vi "DAE Radau 5th Order (VIRef).vi"(5 "data":variant, 7 "DAE F(X,X',t)":refnum<vi>, 8 "error in (no error)":errorcluster, 9 "simulation parameters":T1={"initial time"=0.0, "final time"=10.0, "Absolute Tolerance"=[0.001], "Relative Tolerance"=[0.001], "minimum time step"=1e-08, "maximum time step"=1.0, "initial time step"=0.01} {"initial time step" min=0.0; "maximum time step" min=0.0; "minimum time step" min=0.0}, 10 "Initial Derivatives":dbl[](array[numeric]), 11 "Initial Values":dbl[](array[numeric])) -> (0 "error out":errorcluster, 1 "X Derivatives":dbl[][](array[numeric]), 2 "X Values":dbl[][](array[numeric]), 3 "Times":dbl[](array[numeric]))   [LabVIEW 2020, in "NI_DAE.lvlib"]
doc: "Solves differential algebraic equations (DAEs) with initial conditions by using the Radau IIA method. You must manually select the polymorphic instance to use."
uses:
  <vilib>/gmath/NI_DAE.lvlib
  <vilib>/gmath/dae.llb/Radau5_Parameters.ctl
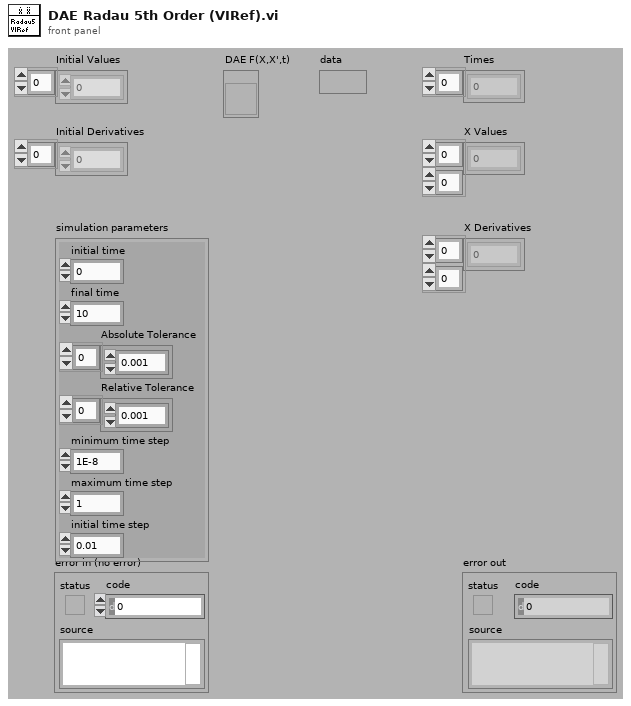
[diagram p1: front panel]
types:
  T1 = typedef "NI_DAE.lvlib/Radau5_Parameters.ctl" = cluster{"initial time":dbl, "final time":dbl, "Absolute Tolerance":dbl[], "Relative Tolerance":dbl[], "minimum time step":dbl, "maximum time step":dbl, "initial time step":dbl}
  T2 = typedef "NI_DAE.lvlib/Radau5_Simulation Data.ctl" = cluster{"initial time":dbl, "final time":dbl, "step size":dbl, "proposed step size":dbl, "max step size":dbl, "min step size":dbl, "Output of T":dbl, "Substep Index":i32, "Timestep Index":i32, "Width":i32, "Absolute tolerance":dbl[], "Relative tolerance":dbl[], "Outputs of Y":dbl[], "Outputs of Y'":dbl[], "Delta":dbl[], "DAE methods":enum16{"default", "Radau IIA"}, "Diag Eval Stage":T3, "step accepted?":bool, "step complete?":bool, "NaN and Inf check?":bool, "First Substep?":bool, "Allow reverse?":bool, "error":errorcluster, "User Jac func?":bool, "Variant":variant, "Index of Y":i8[]}
  T3 = typedef "NI_DAE.lvlib/Radau5_Diag Eval Stage.ctl" = enum16{"Init", "Running", "Final", "End"}
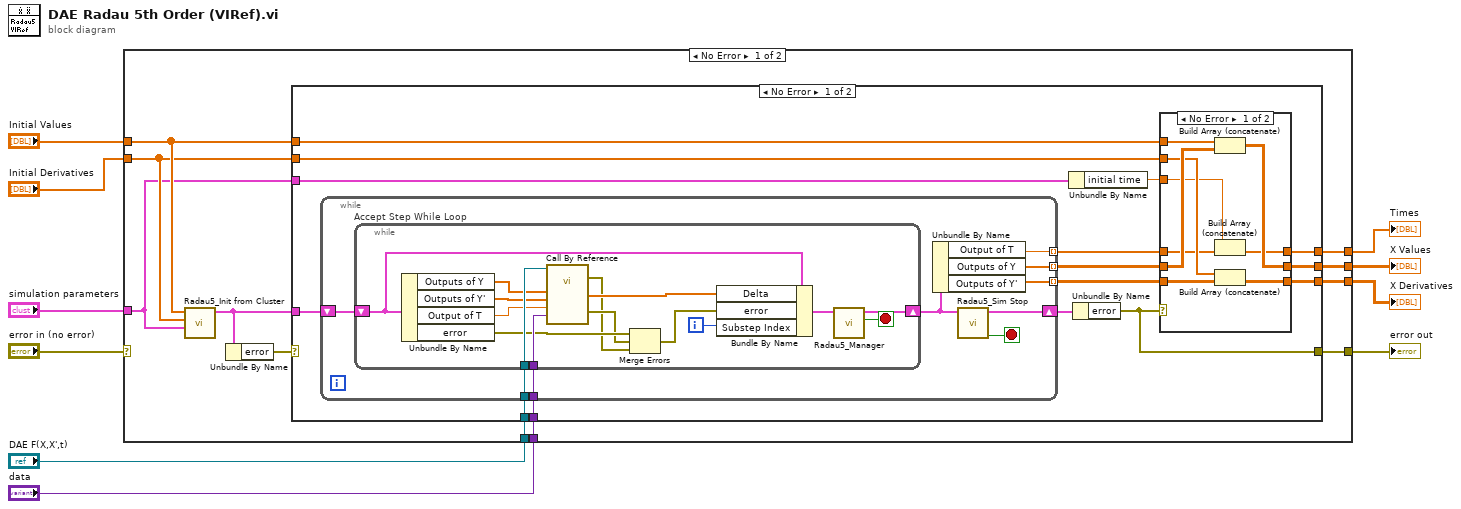
[diagram p0: block diagram]
diagram:
  n1 = case shown="No Error" "error in (no error)" {
    selector: "error in (no error)" -> [_ w71]
    tunnel: [w19 w71] -> w10
    tunnel: [w15 _] -> w9
    tunnel: [w14 _] -> w8
    tunnel: "DAE F(X,X',t)" -> [w21 _]
    tunnel: "data" -> [w20 _]
    tunnel: "Initial Derivatives" -> [w17 _]
    tunnel: "Initial Values" -> [w18 _]
    tunnel: "simulation parameters" -> [w11 _]
    tunnel: [w16 _] -> w1
    frame No Error {
      n2 = call <vilib>:"Radau5_Init from Cluster.vi"("Radau5 Parameters"=w11, "Initial Value Y'"=w17, "Initial Value Y"=w18) -> ("Simulation Data"=w13:T2)  [unwired: 8 in]
      n3 = Unbundle By Name(w13) -> ("error"=w12:errorcluster)
      n4 = case shown="No Error" w12 {
        selector: w12 -> [_ w70]
        tunnel: w21 -> [w35 _]
        tunnel: w20 -> [w34 _]
        tunnel: [w33 w70] -> w19
        tunnel: w18 -> [w29 _]
        tunnel: w17 -> [w28 _]
        tunnel: [w27 _] -> w16
        tunnel: [w26 _] -> w15
        tunnel: [w25 _] -> w14
        tunnel: w13 -> [w24 _]
        tunnel: w11 -> [w23 _]
        frame No Error {
          n5 = while {
            shift-right: [w52] -> w36
            shift-left: w24 -> [w54]
            tunnel: w35 -> [w53]
            tunnel: [w50] -> w30 mode=indexing
            tunnel: [w47] -> w31 mode=indexing
            tunnel: [w49] -> w32 mode=indexing
            tunnel: w34 -> [w46]
            stop <- w51 stop-if-true
            n6 = while "Accept Step While Loop" {
              tunnel: w53 -> [w69]
              shift-right: [w66] -> w48
              shift-left: w54 -> [w68]
              tunnel: w46 -> [w62]
              i -> [w64]
              stop <- w63 stop-if-true
              n7 = Unbundle By Name(w68) -> ("Outputs of Y"=w61:dbl[], "Outputs of Y'"=w60:dbl[], "Output of T"=w59:dbl, "error"=w57:errorcluster)
              n8 = call-by-ref "?"(reference=w69, "data"=w62, "t"=w59, "X'"=w60, "X"=w61) -> (error out=w55:errorcluster, 0:"error out"=w56:errorcluster, "F(X,X',t)"=w65:dbl[])  [unwired: 1 in, 1 out]
              n9 = Merge Errors(w57, w56, w55) -> (w58:errorcluster)
              n10 = Bundle By Name(cluster=w68, "Delta"=w65, "error"=w58, "Substep Index"=w64) -> (w67:T2)
              n11 = call <vilib>:"Radau5_Manager.vi"("Simulation Data In"=w67) -> ("step complete?"=w63:bool, "Simulation Data Out"=w66:T2)  [unwired: 9 in]
            }
            n12 = Unbundle By Name(w48) -> ("Output of T"=w50:dbl, "Outputs of Y"=w47:dbl[], "Outputs of Y'"=w49:dbl[])
            n13 = call <vilib>:"Radau5_Sim Stop.vi"("Simulation Data In"=w48) -> ("Stop simulation?"=w51:bool, "Simulation Data Out"=w52:T2)  [unwired: 9 in]
          }
          n14 = Unbundle By Name(w23) -> ("initial time"=w22:dbl)
          n15 = Unbundle By Name(w36) -> ("error"=w33:errorcluster)
          n16 = case shown="No Error" w33 {
            tunnel: w32 -> [w43 _]
            tunnel: w31 -> [w45 _]
            tunnel: w30 -> [w41 _]
            tunnel: w29 -> [w44 _]
            tunnel: w28 -> [w42 _]
            tunnel: [w40 _] -> w26
            tunnel: [w39 _] -> w27
            tunnel: [w38 _] -> w25
            tunnel: w22 -> [w37 _]
            frame No Error {
              n17 = Build Array (concatenate)(w44, w45) -> (w40:dbl[][])
              n18 = Build Array (concatenate)(w37, w41) -> (w39:dbl[])
              n19 = Build Array (concatenate)(w42, w43) -> (w38:dbl[][])
            }
            frame Error {
            }
          }
        }
        frame Error {
        }
      }
    }
    frame Error {
    }
  }
  "Times" <- w1
  "X Values" <- w9
  "X Derivatives" <- w8
  "error out" <- w10
